vi "SCM.vi"(8 "Stopp":bool, 10 "SLOT":i32 min=0 max=999 step=100 format="%03d", 11 "USB":i32) -> ()   [LabVIEW 2020]
doc: "This VI provides a GUI for SCM modules. It implements an abstract module interface, where callers provide the only necessary and sufficient information for callee modules via the datafields USB, SLOT and Stopp. All module intern information are handled hidden by the module. Thereby, a caller must not \"know\" about such internals."
panel:
  in  "Laser Soft Lock":bool
  out "Laser Locked":bool
  out "Laser Active":bool
  out "Power":bool
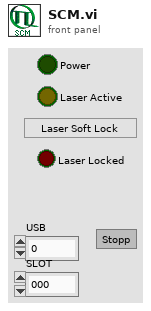
[diagram p1: front panel]
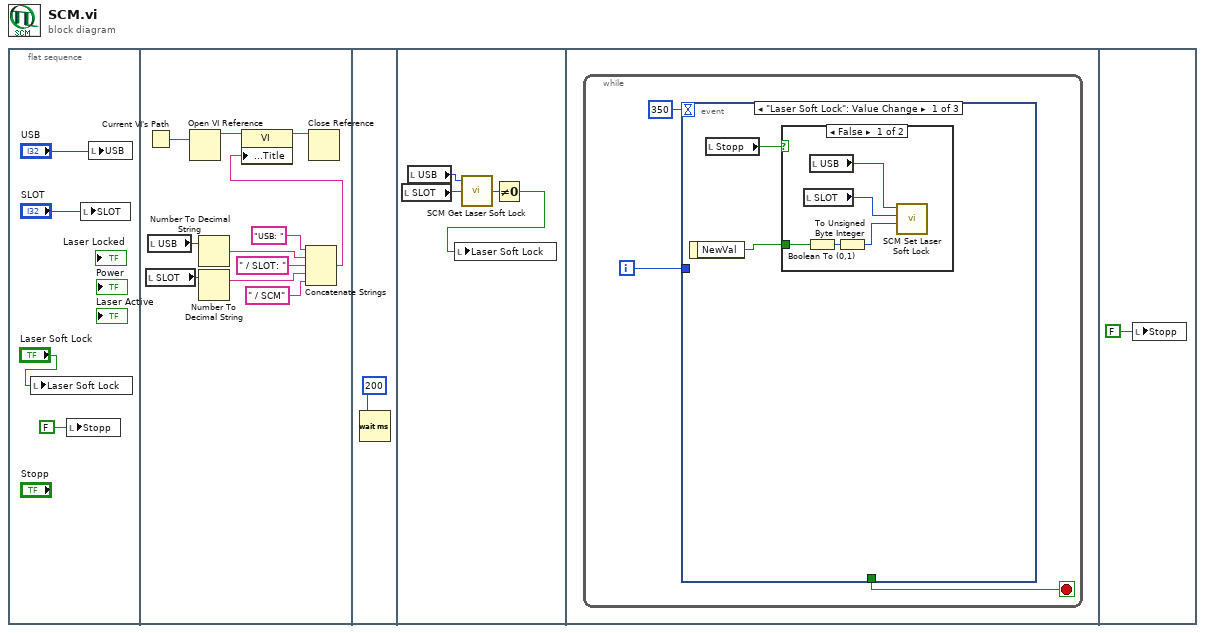
[diagram p0: block diagram]
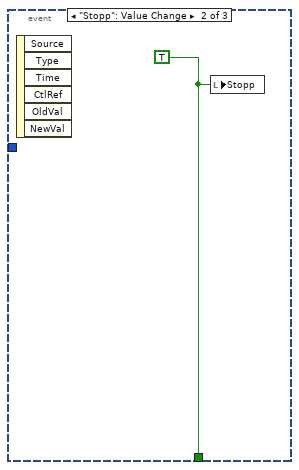
[diagram p3: hidden frame]
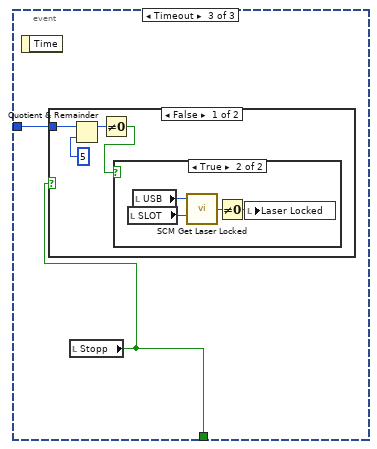
[diagram p4: hidden frame]
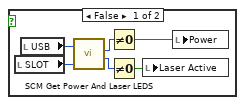
[diagram p5: hidden frame]
diagram:
  n1 = flat-sequence {
    frame #0 {
      n2 = local write "Laser Soft Lock"("Laser Soft Lock") -> ()
      n3 = local write "Stopp"(FALSE ("Stopp")) -> ()
      n4 = local write "SLOT"("SLOT") -> ()
      n5 = local write "USB"("USB") -> ()
    }
    frame #1 {
      n6 = Current VI's Path() -> (path=w13:path)
      n7 = local read "SLOT"() -> (w8:i32)
      n8 = local read "USB"() -> (w11:i32)
      n9 = Open VI Reference(vi path=w13) -> (vi reference=w15:refnum<vi>)  [unwired: 5 in, 1 out]
      n10 = Number To Decimal String(number=w11) -> (decimal integer string=w10:string)  [unwired: 1 in]
      n11 = Number To Decimal String(number=w8) -> (decimal integer string=w7:string)  [unwired: 1 in]
      n12 = Concatenate Strings("USB: " ("Front Panel Window:Title"), w10, " / SLOT: " ("string"), w7, " / SCM" ("string")) -> (w5:string)
      n13 = property class="VI"(reference=w15, "Front Panel.Title"=w5) -> (reference out=w14:refnum<vi>)  [unwired: 1 in, 1 out]
      n14 = Close Reference(reference=w14) -> ()  [unwired: 1 in, 1 out]
    }
    frame #2 {
      n15 = Wait (ms)(milliseconds to wait=200) -> ()  [unwired: 1 out]
    }
    frame #3 {
      n16 = local read "SLOT"() -> (w17:i32)
      n17 = local read "USB"() -> (w18:i32)
      n18 = call "SCM Get Laser Soft Lock.vi"("SlotId"=w17, "DevIdx"=w18) -> ("SoftLocked"=w20:enum8{"SoftLock off", "SoftLock on"})  [unwired: 1 in, 2 out]
      n19 = Not Equal To 0?(x=w20) -> (x != 0?=w19:bool)
      n20 = local write "Laser Soft Lock"(w19) -> ()
    }
    frame #4 {
      n21 = while {
        i -> [w21]
        stop <- w23 stop-if-true
        n22 = event shown="[0] \"Laser Soft Lock\": Value Change" {
          selector: _ -> [_ _ _]
          dyn-events: _ -> [_ _ _]
          timeout: 350 -> [_ _ _]
          tunnel: [_ w31 w32] -> w23
          tunnel: w21 -> [_ _ w33]
          event "Laser Soft Lock": Value Change {
            n23 = event-data() -> ("NewVal"=w25:bool)  [unwired: 1 in]
            n24 = local read "Stopp"() -> (w24:bool)
            n25 = case shown="False" w24 {
              tunnel: w25 -> [w26 _]
              frame False {
                n26 = local read "SLOT"() -> (w27:i32)
                n27 = Boolean To (0,1)(Boolean=w26) -> (0, 1=w29:i16)
                n28 = local read "USB"() -> (w28:i32)
                n29 = To Unsigned Byte Integer(number=w29) -> (unsigned 8bit integer=w30:u8)
                n30 = call "SCM Set Laser Soft Lock.vi"("SoftLock"=w30, "SlotId"=w27, "DevIdx"=w28) -> ()  [unwired: 1 in, 2 out]
              }
              frame True {
              }
            }
          }
          event "Stopp": Value Change {
            w31 = TRUE ("Value (Signaling)")
            n31 = event-data() -> ()  [unwired: 1 in, 6 out]
            n32 = local write "Stopp"(w31) -> ()
          }
          event Timeout {
            n33 = event-data() -> ()  [unwired: 1 in, 1 out]
            n34 = local read "Stopp"() -> (w32:bool)
            n35 = case shown="False" w32 {
              tunnel: w33 -> [w34 _]
              frame False {
                n36 = Quotient & Remainder(x=w34, y=5) -> (x-y*floor(x/y)=w37:i32)  [unwired: 1 out]
                n37 = Not Equal To 0?(x=w37) -> (x != 0?=w36:bool)
                n38 = case shown="True" w36 {
                  frame False {
                    n39 = local read "SLOT"() -> (w42:i32)
                    n40 = local read "USB"() -> (w40:i32)
                    n41 = call "SCM Get Power And Laser LEDS.vi"("DevIdx"=w40, "SlotId"=w42) -> ("PowerLED"=w41:u8, "LaserActiveLED"=w43:u8)  [unwired: 1 in, 2 out]
                    n42 = Not Equal To 0?(x=w41) -> (x != 0?=w39:bool)
                    n43 = Not Equal To 0?(x=w43) -> (x != 0?=w38:bool)
                    n44 = local write "Laser Active"(w38) -> ()
                    n45 = local write "Power"(w39) -> ()
                  }
                  frame True {
                    n46 = local read "SLOT"() -> (w46:i32)
                    n47 = local read "USB"() -> (w45:i32)
                    n48 = call "SCM Get Laser Locked.vi"("SlotId"=w46, "DevIdx"=w45) -> ("LaserLocked"=w47:enum8{"Laser unlocked", "Laser locked"})  [unwired: 1 in, 2 out]
                    n49 = Not Equal To 0?(x=w47) -> (x != 0?=w44:bool)
                    n50 = local write "Laser Locked"(w44) -> ()
                  }
                }
              }
              frame True {
              }
            }
          }
        }
      }
    }
    frame #5 {
      n51 = local write "Stopp"(FALSE ("Stopp")) -> ()
    }
  }
